vi "Word_Set_Chart_Axis_Font.vi"(0 "Word.InlineShapes":refnum<k7>, 5 "Type":i32(ring)=1 items=["xlCategory"=1, "xlSeriesAxis"=3, "xlValue"=2], 7 "number format":string, 9 "Chart index":i16=-1, 11 "error in":errorcluster, 12 "axis font":T1={"font style"="", "bold"=FALSE, "italic"=FALSE, "underline"=FALSE, "size"=10.0, "color"=4278190080} {"size" format="%.2f"}, 13 "title":string) -> (15 "error out":errorcluster)   [LabVIEW 2017, in "NI_ReportGenerationToolkit.lvlib"]
uses:
  <vilib>/addons/_office/NI_ReportGenerationToolkit.lvlib
panel:
  in  "Graph.Axes":refnum<k7>
  in  "Graph.Chart":refnum<k7>
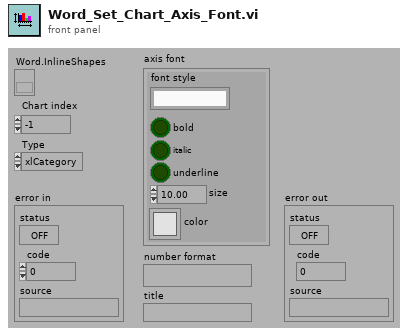
[diagram p1: front panel]
types:
  T1 = cluster{"font style":string, "bold":bool, "italic":bool, "underline":bool, "size":sgl, "color":u32}
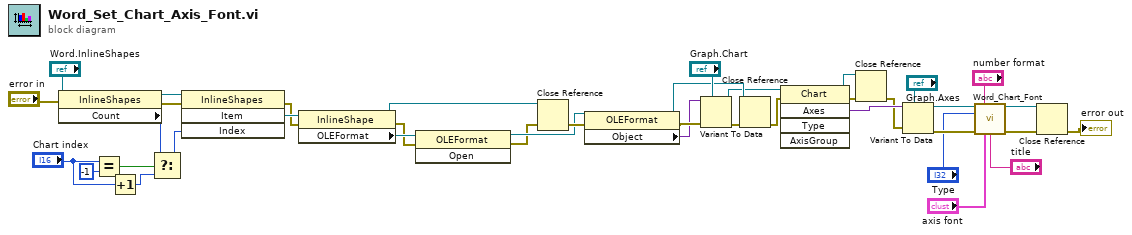
[diagram p0: block diagram]
diagram:
  n1 = property class="InlineShapes"(reference="Word.InlineShapes", error in="error in") -> (reference out=w27:refnum<k7>, error out=w38:errorcluster, "Count"=w22:i32)
  n2 = Equal?(x="Chart index", y=i16 -1) -> (x = y?=w26:bool)
  n3 = Increment(x="Chart index") -> (x+1=w24:i16)
  n4 = Select(t=w22, s=w26, f=w24) -> (s? t:f=w21:i32)
  n5 = invoke class="InlineShapes" method="Item"(reference=w27, error in=w38, "Index"=w21) -> (error out=w29:errorcluster, "Item"=w30:refnum<k7>)  [unwired: 1 in, 2 out]
  n6 = property class="InlineShape"(reference=w30, error in=w29) -> (reference out=w33:refnum<k7>, error out=w2:errorcluster, "OLEFormat"=w4:refnum<k7>)
  n7 = invoke class="OLEFormat" method="Open"(reference=w4, error in=w2) -> (reference out=w3:refnum<k7>, error out=w1:errorcluster)  [unwired: 1 in, 1 out]
  n8 = Close Reference(reference=w33, error in (no error)=w1) -> (error out=w32:errorcluster)
  n9 = property class="OLEFormat"(reference=w3, error in=w32) -> (reference out=w31:refnum<k7>, error out=w37:errorcluster, "Object"=w36:variant)
  n10 = Variant To Data(error in=w37, type="Graph.Chart", Variant=w36) -> (data=w20:refnum<k7>, error out=w34:errorcluster)
  n11 = Close Reference(reference=w31, error in (no error)=w34) -> (error out=w19:errorcluster)
  n12 = invoke class="Chart" method="Axes"(reference=w20, error in=w19) -> (reference out=w14:refnum<k7>, error out=w15:errorcluster, "Axes"=w17:variant)  [unwired: 3 in, 2 out]
  n13 = Close Reference(reference=w14, error in (no error)=w15) -> (error out=w16:errorcluster)
  n14 = Variant To Data(error in=w16, type="Graph.Axes", Variant=w17) -> (data=w10:refnum<k7>, error out=w9:errorcluster)
  n15 = call <vilib>:"Word_Chart_Font.vi"("axes in"=w10, "number format"="number format", "type"="Type", "error in"=w9, "axis font"="axis font", "title"="title") -> ("axes out"=w11:refnum<k7>, "error out"=w12:errorcluster)  [unwired: 8 out]
  n16 = Close Reference(reference=w11, error in (no error)=w12) -> (error out=→"error out":errorcluster)
